vi "0mqPubRep.vi"(10 "intercomm configuration":T1) -> (0 "last error":errorcluster, 1 "exit":bool)   [LabVIEW 2018]
uses:
  Custom/S4msg.ctl
  <vilib>/addons/zeromq/socket_type.ctl
  <vilib>/addons/zeromq/zeromq.lvlib
  <vilib>/addons/zeromq/zmq_context.lvclass
  <vilib>/addons/zeromq/zmq_socket.lvclass
panel:
  out "stopped":bool
  out "endpointREP":string="localhost"
  out "last tick":u32
  out "endpointPUB":string="localhost"
  out "S4ICS_status":string caption="Status received from S4ICS"
  out "S4ICS_command":string caption="Command sent to S4ICS"
  in  "Stop Client":bool
  # "S4ICS 0mqPubRep"
  # "COMMUNICATION CHANNEL"
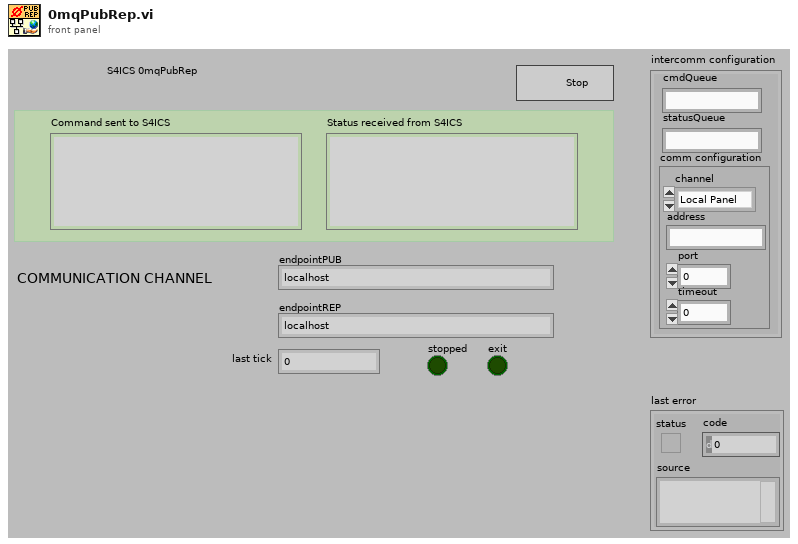
[diagram p1: front panel]
types:
  T1 = cluster{"S4commandQueueName":string, "S4statusQueueName":string, "comm configuration":cluster{"channel":enum32{"Local Panel", "Inner TCP/IP", "Outer TCP/IP", "MQTT", "ZeroMQ"}, "address":string, "port":u16, "timeout":i32}}
  T2 = typedef "zeromq.lvlib/socket_type.ctl" = enum8{"ZMQ_PAIR", "ZMQ_PUB", "ZMQ_SUB", "ZMQ_REQ", "ZMQ_REP", "ZMQ_DEALER", "ZMQ_ROUTER", "ZMQ_PULL", "ZMQ_PUSH", "ZMQ_XPUB", "ZMQ_XSUB", "ZMQ_STREAM", "ZMQ_SERVER", "ZMQ_CLIENT", "ZMQ_RADIO", "ZMQ_DISH", "ZMQ_GATHER", "ZMQ_SCATTER", "ZMQ_DGRAM"}
  T3 = typedef "S4msg.ctl" = cluster{"msg topic":string, "msg data":variant}
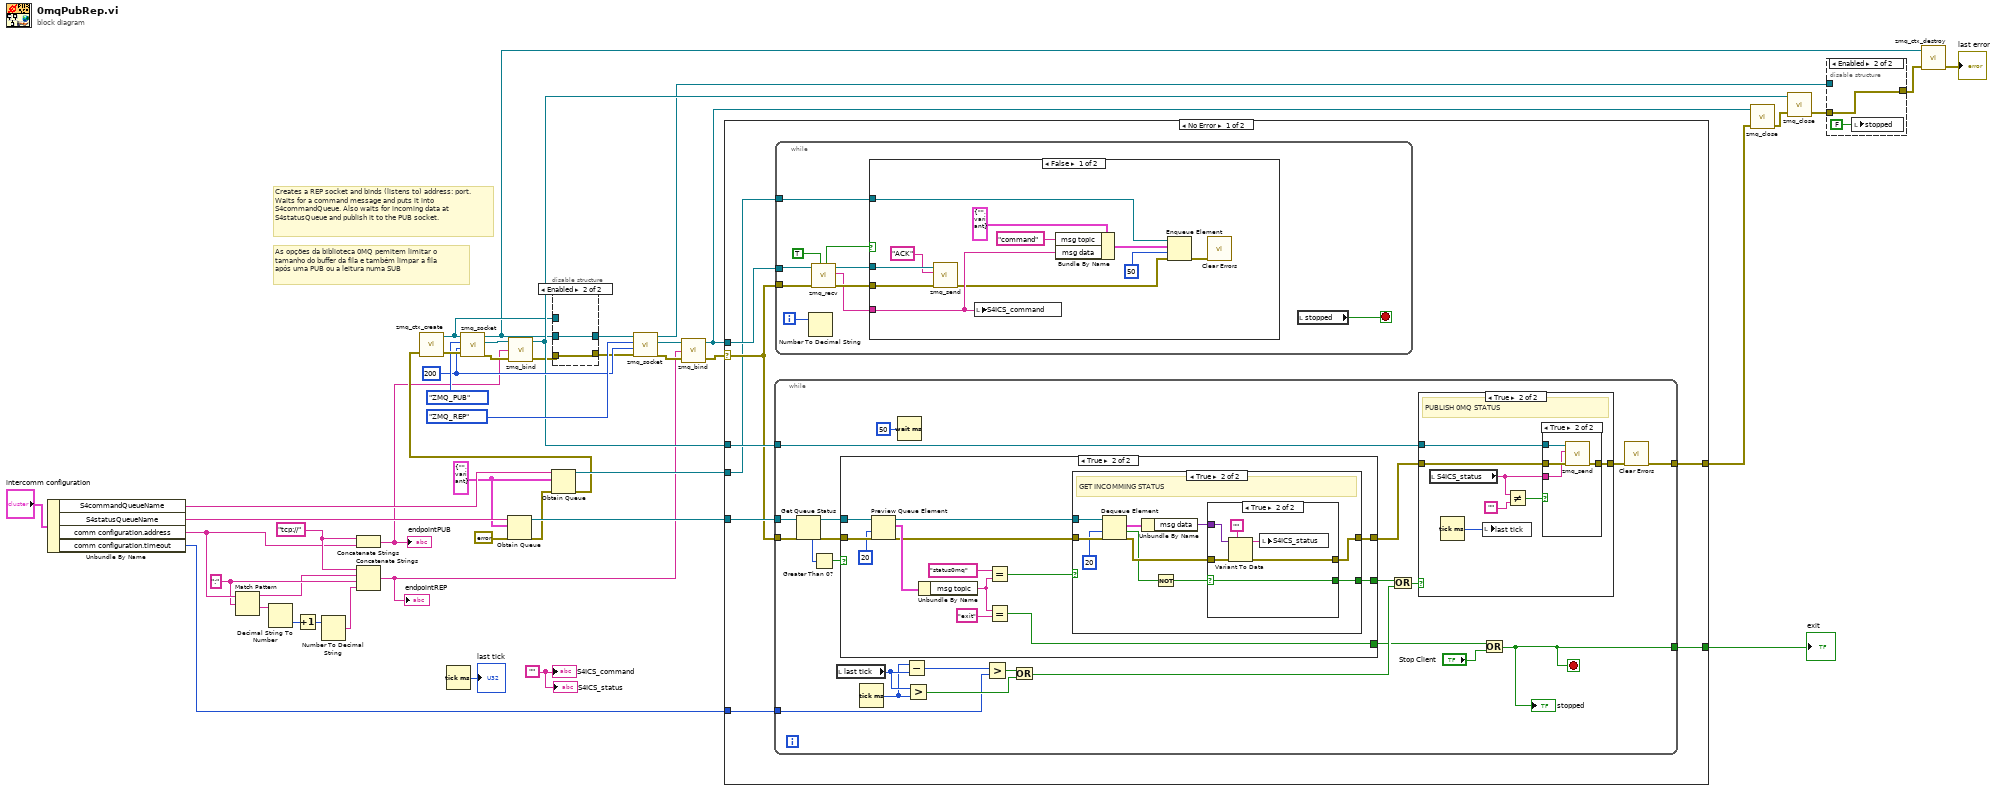
[diagram p0: block diagram]
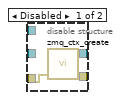
[diagram p2: hidden frame]
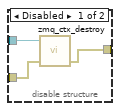
[diagram p3: hidden frame]
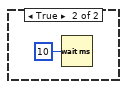
[diagram p4: hidden frame]
diagram:
  w6 = ":"
  w10 = "tcp://"
  w27 = 200 ("linger (ms)")
  w37 = T3 {"msg topic"="", "msg data"=variant} ("S4msg")
  w45 = ""
  # "As opções da biblioteca 0MQ pemitem limitar o tamanho do buffer da fila e também limpar a fila após uma PUB ou a leitura numa SUB"
  # "Creates a REP socket and binds (listens to) address: port. Waits for a command message and puts it into S4commandQueue. Also waits for incoming data at S4statusQueue and publish it to the PUB socket."
  n1 = Unbundle By Name("intercomm configuration") -> ("S4commandQueueName"=w43:string, "S4statusQueueName"=w44:string, "comm configuration.address"=w7:string, "comm configuration.timeout"=w23:i32)
  n2 = Match Pattern(string=w7, regular expression=w6) -> (before substring=w2:string, after substring=w5:string)  [unwired: 1 in, 2 out]
  n3 = Decimal String To Number(string=w5) -> (number=w4:i32)  [unwired: 2 in, 1 out]
  n4 = Increment(x=w4) -> (x+1=w3:i32)
  n5 = Number To Decimal String(number=w3) -> (decimal integer string=w1:string)  [unwired: 1 in]
  n6 = Concatenate Strings(w10, w7) -> (w9:string)
  "endpointPUB" <- w9
  n7 = Concatenate Strings(w10, w2, w6, w1) -> (w8:string)
  "endpointREP" <- w8
  n8 = Tick Count (ms)() -> (millisecond timer value=→"last tick":u32)
  n9 = Obtain Queue(name (unnamed)=w44, element data type=w37, error in (no error)=errorcluster {"status"=FALSE, "code"=0, "source"=""}) -> (queue out=w41:refnum<queue>, error out=w38:errorcluster)  [unwired: 2 in, 1 out]
  n10 = Obtain Queue(name (unnamed)=w43, element data type=w37, error in (no error)=w38) -> (queue out=w42:refnum<queue>, error out=w40:errorcluster)  [unwired: 2 in, 1 out]
  n11 = call <vilib>:"zmq_ctx_create.vi"("error in"=w40) -> ("error out"=w35:errorcluster, "context out"=w12:refnum<class "zmq_context.lvclass">)  [unwired: 3 in]
  n12 = call <vilib>:"zmq_socket.vi"("error in"=w35, "linger (ms)"=w27, "socket type"=socket_type."ZMQ_PUB", "context in"=w12) -> ("error out"=w36:errorcluster, "socket out"=w33:refnum<class "zmq_socket.lvclass">, "context out"=w11:refnum<class "zmq_context.lvclass">)  [unwired: 1 in]
  n13 = call <vilib>:"zmq_bind.vi"("error in"=w36, "endpoint"=w9, "socket in"=w33) -> ("error out"=w15:errorcluster, "socket out"=w20:refnum<class "zmq_socket.lvclass">)  [unwired: 1 in]
  n14 = disable-structure shown="Enabled" {
    disable-tunnel: [w48 w49] -> w16
    disable-tunnel: w15 -> [w47 w50]
    disable-tunnel: [w46 w50] -> w14
    disable-tunnel: w12 -> [_ _]
    disable-tunnel: w11 -> [_ w49]
    frame Disabled {
      n15 = call <vilib>:"zmq_ctx_create.vi"("error in"=w47) -> ("error out"=w46:errorcluster, "context out"=w48:refnum<class "zmq_context.lvclass">)  [unwired: 3 in]
    }
    frame Enabled {
    }
  }
  n16 = call <vilib>:"zmq_socket.vi"("error in"=w14, "linger (ms)"=w27, "socket type"=socket_type."ZMQ_REP", "context in"=w16) -> ("error out"=w32:errorcluster, "socket out"=w30:refnum<class "zmq_socket.lvclass">, "context out"=w18:refnum<class "zmq_context.lvclass">)  [unwired: 1 in]
  n17 = call <vilib>:"zmq_bind.vi"("error in"=w32, "endpoint"=w8, "socket in"=w30) -> ("error out"=w26:errorcluster, "socket out"=w24:refnum<class "zmq_socket.lvclass">)  [unwired: 1 in]
  n18 = case shown="No Error" w26 {
    selector: w26 -> [w52 w152]
    tunnel: w42 -> [w51 _]
    tunnel: w41 -> [w58 _]
    tunnel: w24 -> [w53 _]
    tunnel: w20 -> [w57 _]
    tunnel: [w56 w152] -> w25
    tunnel: w23 -> [w55 _]
    tunnel: [w54 _] -> w13
    frame No Error {
      n19 = while {
        tunnel: [w90] -> w56
        tunnel: w58 -> [w103]
        tunnel: w57 -> [w95]
        tunnel: w52 -> [w91]
        tunnel: w55 -> [w88]
        tunnel: [w83] -> w54
        stop <- w83 stop-if-true
        n20 = Get Queue Status(queue=w103, error in (no error)=w91) -> (queue out=w87:refnum<queue>, error out=w86:errorcluster, # elements in queue=w84:i32)  [unwired: 1 in, 5 out]
        n21 = Greater Than 0?(x=w84) -> (x > 0?=w85:bool)
        n22 = local read "last tick"() -> (w101:u32)
        n23 = case shown="True" w85 {
          selector: w85 -> [w104 _]
          tunnel: [w105 w118] -> w94
          tunnel: [w104 w117] -> w92
          tunnel: [w104 w106] -> w89
          tunnel: w87 -> [_ w116]
          tunnel: w86 -> [w105 w115]
          frame False {
          }
          frame True {
            n24 = Preview Queue Element(queue=w116, timeout in ms (-1)=20, error in (no error)=w115) -> (queue out=w111:refnum<queue>, element=w114:T3, error out=w110:errorcluster)  [unwired: 1 out]
            n25 = Unbundle By Name(w114) -> ("msg topic"=w107:string)
            n26 = Equal?(x="status0mq" ("msg topic"), y=w107) -> (x = y?=w112:bool)
            n27 = Equal?(x=w107, y="exit" ("msg topic")) -> (x = y?=w106:bool)
            n28 = case shown="True" w112 {
              selector: w112 -> [w119 _]
              tunnel: w110 -> [w120 w130]
              tunnel: w111 -> [_ w129]
              tunnel: [w120 w125] -> w118
              tunnel: [w119 w121] -> w117
              frame False {
              }
              frame True {
                # "GET INCOMMING STATUS"
                n29 = Dequeue Element(queue=w129, timeout in ms (-1)=20, error in (no error)=w130) -> (element=w128:T3, timed out?=w123:bool, error out=w126:errorcluster)  [unwired: 1 out]
                n30 = Unbundle By Name(w128) -> ("msg data"=w127:variant)
                n31 = Not(x=w123) -> (.not. x?=w122:bool)
                n32 = case shown="True" w122 {
                  selector: w122 -> [w132 w133]
                  tunnel: w127 -> [_ w138]
                  tunnel: w126 -> [w131 w137]
                  tunnel: [w131 w136] -> w125
                  tunnel: [w132 w133] -> w121
                  frame False {
                  }
                  frame True {
                    n33 = Variant To Data(error in=w137, type="", Variant=w138) -> (data=w134:string, error out=w136:errorcluster)
                    n34 = local write "S4ICS_status"(w134) -> ()
                  }
                }
              }
            }
          }
        }
        n35 = Tick Count (ms)() -> (millisecond timer value=w100:u32)
        n36 = Wait (ms)(milliseconds to wait=u32 50) -> ()  [unwired: 1 out]
        n37 = Subtract(x=w100, y=w101) -> (x-y=w102:u32)
        n38 = Greater?(x=w101, y=w100) -> (0:w98:bool)
        n39 = Greater?(x=w102, y=w88) -> (0:w99:bool)
        n40 = Or(x=w99, y=w98) -> (x .or. y?=w97:bool)
        n41 = Or(x=w92, y=w97) -> (x .or. y?=w96:bool)
        n42 = case shown="True" w96 {
          tunnel: [w139 w143] -> w93
          tunnel: w95 -> [_ w146]
          tunnel: w94 -> [w139 w145]
          frame False {
          }
          frame True {
            # "PUBLISH 0MQ STATUS"
            n43 = local read "S4ICS_status"() -> (w140:string)
            n44 = Tick Count (ms)() -> (millisecond timer value=w144:u32)
            n45 = local write "last tick"(w144) -> ()
            n46 = Not Equal?(x=w140, y="") -> (x != y?=w141:bool)
            n47 = case shown="True" w141 {
              tunnel: w146 -> [_ w151]
              tunnel: w145 -> [w147 w150]
              tunnel: [w147 w149] -> w143
              tunnel: w140 -> [_ w148]
              frame False {
              }
              frame True {
                n48 = call <vilib>:"zmq_send.vi"("error in"=w150, "data"=w148, "socket in"=w151) -> ("error out"=w149:errorcluster)  [unwired: 4 in, 1 out]
              }
            }
          }
        }
        n49 = Or(x=w89, y="Stop Client") -> (x .or. y?=w83:bool)
        "stopped" <- w83
        n50 = call <vilib>:"Clear Errors.vi"("error in (no error)"=w93) -> ("error out"=w90:errorcluster)  [unwired: 5 in, 1 out]
      }
      n51 = while {
        tunnel: w53 -> [w67]
        tunnel: w52 -> [w68]
        tunnel: w51 -> [w59]
        i -> [w64]
        stop <- w61 stop-if-true
        n52 = Number To Decimal String(number=w64) -> ()  [unwired: 1 in, 1 out]
        n53 = call <vilib>:"zmq_recv.vi"("no block? (F)"=TRUE, "error in"=w68, "socket in"=w67) -> ("error out"=w66:errorcluster, "data"=w60:string, "socket out"=w65:refnum<class "zmq_socket.lvclass">, "timeout?"=w62:bool)  [unwired: 2 in, 1 out]
        n54 = case shown="False" w62 {
          tunnel: w66 -> [w79 _]
          tunnel: w65 -> [w78 _]
          tunnel: w60 -> [w71 _]
          tunnel: w59 -> [w69 _]
          frame False {
            n55 = call <vilib>:"zmq_send.vi"("error in"=w79, "data"="ACK", "socket in"=w78) -> ("error out"=w70:errorcluster)  [unwired: 4 in, 1 out]
            n56 = local write "S4ICS_command"(w71) -> ()
            n57 = Bundle By Name(cluster=T3 {"msg topic"="", "msg data"=variant} ("S4msg"), "msg topic"="command", "msg data"=w71) -> (w75:T3)
            n58 = Enqueue Element(queue=w69, element=w75, timeout in ms (-1)=50, error in (no error)=w70) -> (error out=w76:errorcluster)  [unwired: 2 out]
            n59 = call <vilib>:"Clear Errors.vi"("error in (no error)"=w76) -> ()  [unwired: 5 in, 2 out]
          }
          frame True {
            n60 = Wait (ms)(milliseconds to wait=u32 10) -> ()  [unwired: 1 out]
          }
        }
        n61 = local read "stopped"() -> (w61:bool)
      }
    }
    frame Error {
    }
  }
  "exit" <- w13
  n62 = call <vilib>:"zmq_close.vi"("error in"=w25, "socket"=w24) -> ("error out"=w22:errorcluster)  [unwired: 3 in]
  n63 = call <vilib>:"zmq_close.vi"("error in"=w22, "socket"=w20) -> ("error out"=w21:errorcluster)  [unwired: 3 in]
  n64 = disable-structure shown="Enabled" {
    disable-tunnel: w21 -> [w155 w157]
    disable-tunnel: [w154 w157] -> w19
    disable-tunnel: w18 -> [w153 _]
    frame Disabled {
      n65 = call <vilib>:"zmq_ctx_destroy.vi"("error in"=w155, "context in"=w153) -> ("error out"=w154:errorcluster)  [unwired: 3 in]
    }
    frame Enabled {
      n66 = local write "stopped"(FALSE) -> ()
    }
  }
  n67 = call <vilib>:"zmq_ctx_destroy.vi"("error in"=w19, "context in"=w11) -> ("error out"=→"last error":errorcluster)  [unwired: 3 in]
  "S4ICS_command" <- w45
  "S4ICS_status" <- w45
